vi "PixPerDegree.vi"(8 "Monitor Resolution":i32, 9 "Resolution":i32, 10 "distance":dbl format="%0.2f", 11 "Monitor Size":dbl format="%0.2f") -> (2 "degrees":dbl, 3 "Pixels/Degree":dbl)   [LabVIEW 2014]
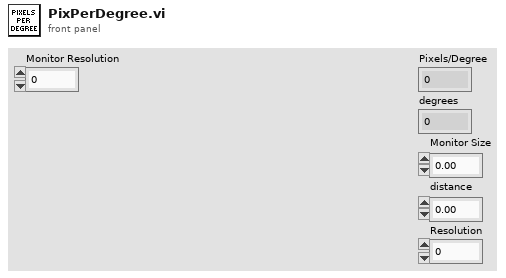
[diagram p1: front panel]
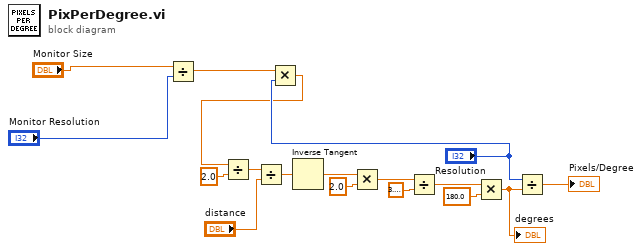
[diagram p0: block diagram]
diagram:
  n1 = Divide(x="Monitor Size", y="Monitor Resolution") -> (x/y=w3:dbl)
  n2 = Multiply(x=w3, y="Resolution") -> (x*y=w1:dbl)
  n3 = Divide(x=w1, y=2.0) -> (x/y=w16:dbl)
  n4 = Divide(x=w16, y="distance") -> (x/y=w14:dbl)
  n5 = Inverse Tangent(1:w14) -> (0:w10:dbl)
  n6 = Multiply(x=w10, y=2.0) -> (x*y=w8:dbl)
  n7 = Divide(x=w8, y=3.141592653589793) -> (x/y=w11:dbl)
  n8 = Multiply(x=w11, y=180.0) -> (x*y=w7:dbl)
  "degrees" <- w7
  n9 = Divide(x="Resolution", y=w7) -> (x/y=→"Pixels/Degree":dbl)
